vi "set_images_per_sweep.vi"(8 "error in (no error)":errorcluster, 10 "images per sweep":i32, 11 "DL090215DataCollection.lvclass in":refnum<class "DataCollectionDL090215.lvclass">) -> (0 "error out":errorcluster, 3 "DL090215DataCollection.lvclass out":refnum<class "DataCollectionDL090215.lvclass">)   [LabVIEW 2010, in "DataCollectionDL090215.lvclass"]
uses:
  DataCollectionDL090215.lvclass
  DataCollectionDL090215.lvclass/DataCollectionDL090215.ctl
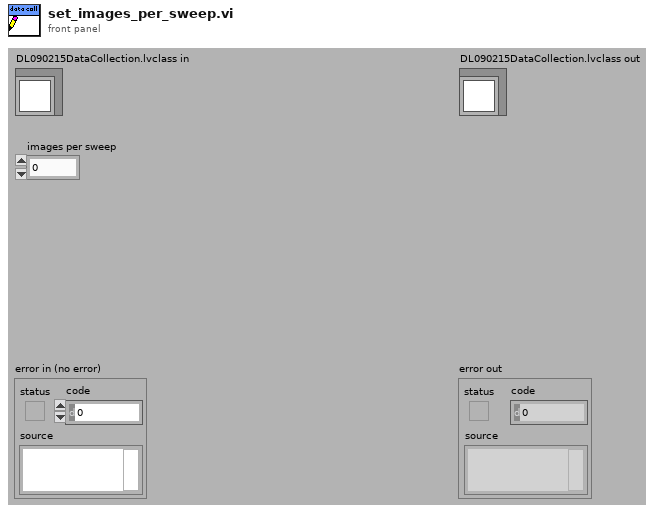
[diagram p1: front panel]
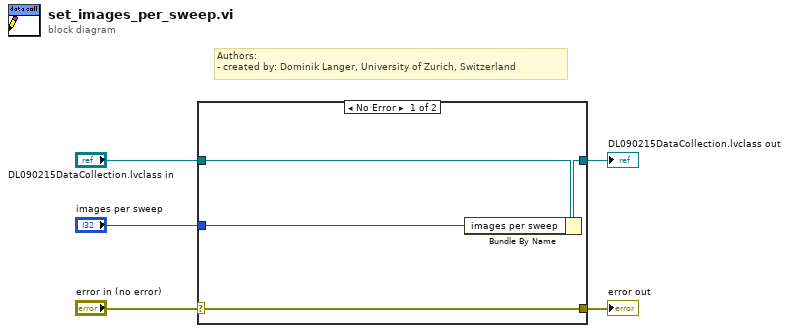
[diagram p0: block diagram]
diagram:
  # "Authors: \n- created by: Dominik Langer, University of Zurich, Switzerland"
  n1 = case shown="No Error" "error in (no error)" {
    selector: "error in (no error)" -> [w9 w10]
    tunnel: [w9 w10] -> w4
    tunnel: [w7 w11] -> w2
    tunnel: "DL090215DataCollection.lvclass in" -> [w8 w11]
    tunnel: "images per sweep" -> [w6 _]
    frame No Error {
      n2 = Bundle By Name(cluster=w8, "images per sweep"=w6) -> (w7:refnum<class "DataCollectionDL090215.lvclass">)
    }
    frame Error {
    }
  }
  "error out" <- w4
  "DL090215DataCollection.lvclass out" <- w2
